vi "testCalcUk.vi"(8 "error in (no error)":errorcluster) -> (0 "error out":errorcluster)   [LabVIEW 2016]
uses:
  ZTAAC/ZTAAC.lvclass
  StrictDef/FilterType.ctl
  StrictDef/InstName.ctl
  <vilib>/Analysis/BLAS.llb/dasum - Absolute Values Sum (DBL).vi
  <vilib>/addons/_JKI Toolkits/Caraya/classes/Test/Test.lvclass
  <vilib>/Analysis/NI_AALBLAS.lvlib
  <vilib>/addons/_JKI Toolkits/Caraya/classes/Assert/Assert.lvclass
panel:
  in  "ZTAAC.lvclass":refnum<class "ZTAAC.lvclass">
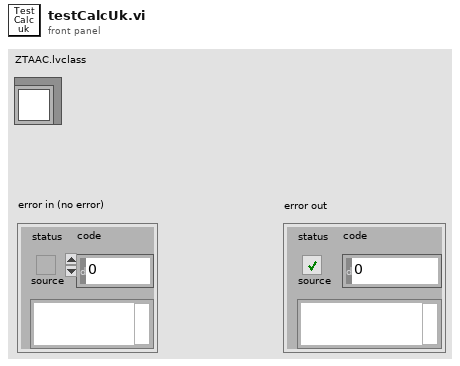
[diagram p1: front panel]
types:
  T1 = typedef "InstName.ctl" = enum16{"lsst", "comcam"}
  T2 = cluster{"Config Dir":path, "Inst Name":T1, "OptStateEsti Config File Name":string, "Mapping File Name":string, "Wavelength Table":string, "Intrinc Zk File Name":string, "y2 Corection File Name":string, "Index DOF File Name":string, "OptCtrl Config File Name":string, "State 0 File Name":string, "Weighting File Name":string, "PSSN Alpha File Name":string, "Authority Files":cluster{"Rigid Body Stroke File":string, "M1M3 Subsystem":cluster{"Mirror":string, "Actuatro Force File":string}, "M2 Subsystem":cluster{"Mirror":string, "Actuatro Force File":string}, "Num of Bending Mode":i32}, "Truncation Threshold":dbl}
  T3 = typedef "FilterType.ctl" = enum16{"ref", "u", "g", "r", "i", "z", "y"}
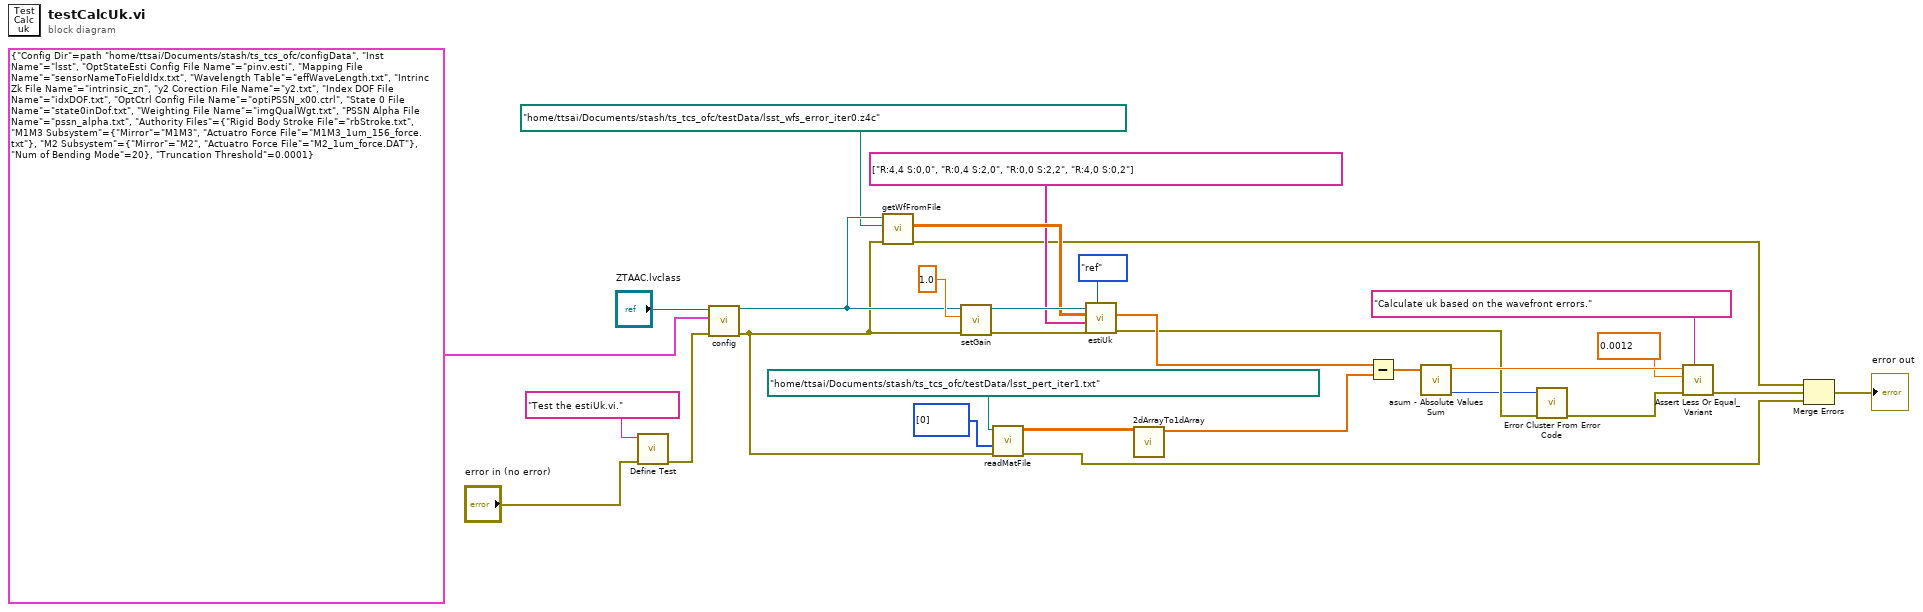
[diagram p0: block diagram]
diagram:
  n1 = call <vilib>:"Define Test.vi"("error in (no error)"="error in (no error)", "Label (VI Title)"="Test the estiUk.vi.") -> ("error out"=w19:errorcluster)  [unwired: 9 in]
  n2 = call "config.vi"("error in (no error)"=w19, "ZTAAC Configuration"=T2 {"Config Dir"=path "/home/ttsai/Documents/stash/ts_tcs_ofc/configData", "Inst Name"=enum."lsst", "OptStateEsti Config File Name"="pinv.esti", "Mapping File Name"="sensorNameToFieldIdx.txt", "Wavelength Table"="effWaveLength.txt", "Intrinc Zk File Name"="intrinsic_zn", "y2 Corection File Name"="y2.txt", "Index DOF File Name"="idxDOF.txt", "OptCtrl Config File Name"="optiPSSN_x00.ctrl", "State 0 File Name"="state0inDof.txt", "Weighting File Name"="imgQualWgt.txt", "PSSN Alpha File Name"="pssn_alpha.txt", "Authority Files"={"Rigid Body Stroke File"="rbStroke.txt", "M1M3 Subsystem"={"Mirror"="M1M3", "Actuatro Force File"="M1M3_1um_156_force.txt"}, "M2 Subsystem"={"Mirror"="M2", "Actuatro Force File"="M2_1um_force.DAT"}, "Num of Bending Mode"=20}, "Truncation Threshold"=0.0001}, "ZTAAC in"="ZTAAC.lvclass") -> ("error out"=w16:errorcluster, "ZTAAC out"=w28:refnum<class "ZTAAC.lvclass">)  [unwired: 7 in]
  n3 = call "getWfFromFile.vi"("error in (no error)"=w16, "Wfs Err Data"=path "/home/ttsai/Documents/stash/ts_tcs_ofc/testData/lsst_wfs_error_iter0.z4c", "ZTAAC in"=w28) -> ("error out"=w15:errorcluster, "Wavefront Error"=w25:dbl[][])  [unwired: 6 in, 1 out]
  n4 = call "setGain.vi"("error in (no error)"=w16, "Gain"=1.0, "ZTAAC in"=w28) -> ("error out"=w17:errorcluster, "ZTAAC out"=w26:refnum<class "ZTAAC.lvclass">)  [unwired: 7 in]
  n5 = call "readMatFile.vi"("error in (no error)"=w16, "Skip Col Idx"=i32[] [0] ("Skip Row Idx"), "Path"=path "/home/ttsai/Documents/stash/ts_tcs_ofc/testData/lsst_pert_iter1.txt" ("Wfs Err Data")) -> ("error out"=w14:errorcluster, "Matrix"=w22:dbl[][])  [unwired: 7 in]
  n6 = call "estiUk.vi"("Filter Type"=FilterType."ref", "error in (no error)"=w17, "Sensor Name"=string[] ["R:4,4 S:0,0", "R:0,4 S:2,0", "R:0,0 S:2,2", "R:4,0 S:0,2"], "Wavefront Error"=w25, "ZTAAC in"=w26) -> ("error out"=w7:errorcluster, "uk Array"=w12:dbl[])  [unwired: 4 in, 1 out]
  n7 = call "2dArrayTo1dArray.vi"("2D Array"=w22) -> ("1D Array"=w11:dbl[])  [unwired: 10 in]
  n8 = Subtract(x=w12, y=w11) -> (x-y=w10:dbl[])
  n9 = call-poly <vilib>:"asum - Absolute Values Sum.vi"("x"=w10) -> ("error"=w6:i32, "dasum"=w9:dbl)  [unwired: 9 in]
  n10 = call <vilib>:"Error Cluster From Error Code.vi"("error in (no error)"=w7, "error code (0)"=w6) -> ("error out"=w5:errorcluster)  [unwired: 7 in]
  n11 = call <vilib>:"Assert Less Or Equal_Variant.vi"("Label"="Calculate uk based on the wavefront errors.", "error in (no error)"=w5, "Y"=0.0012, "X"=w9) -> ("error out"=w4:errorcluster)  [unwired: 7 in]
  n12 = Merge Errors(w15, w4, w14) -> (→"error out":errorcluster)
